vi "dfd_2-band Filter Bank Param Validation.vi"(4 "fs in [Hz]":dbl=800.0, 6 "weight":dbl=0.5, 7 "phase option":u16(ring) items=["Min-Max Phase", "Linear Phase"], 8 "error in (no error)":errorcluster, 9 "stopband attenuation [dB]":dbl=60.0, 10 "roll off":dbl=0.2, 11 "order":i32=38) -> (0 "error out":errorcluster, 1 "dup stopband attenuation [dB]":dbl=60.0, 2 "dup roll off":dbl, 3 "dup order":i32)   [LabVIEW 2017, in "NI_DigFilter_FilterBank.lvlib"]
doc: "Validates the parameters for the prototype filter design. If any parameter is not in their range, this VI will give an error report. If the order is not an integer of 2kM this VI will give a warning report, where k is any positive integer, and M is specified by <B>number of bands</B>."
uses:
  <vilib>/addons/Digital Filter Design/NI_DigFilter_FilterBank.lvlib
  <vilib>/addons/Digital Filter Design/_Misc.llb/dfd_Error Handlers (Multiple).vi
  <vilib>/addons/Digital Filter Design/NI_DigFilterLicensed.lvlib
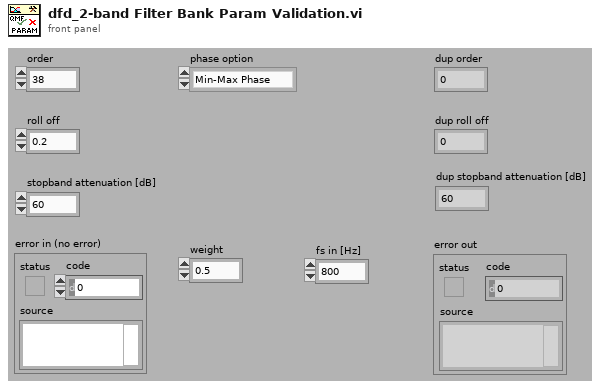
[diagram p1: front panel]
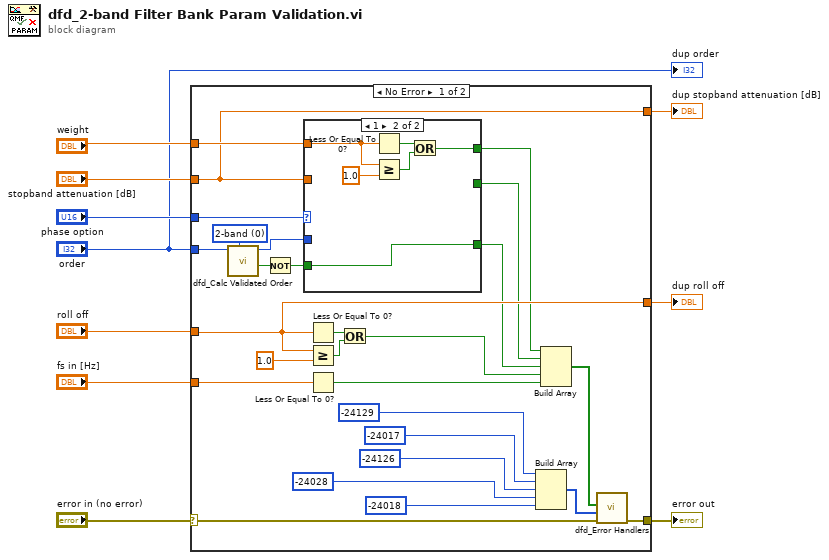
[diagram p0: block diagram]
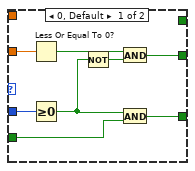
[diagram p2: hidden frame]
diagram:
  n1 = case shown="No Error" "error in (no error)" {
    selector: "error in (no error)" -> [w30 w52]
    tunnel: "order" -> [w15 _]
    tunnel: "roll off" -> [w33 _]
    tunnel: "weight" -> [w27 _]
    tunnel: [w35 w52] -> w8
    tunnel: [w33 _] -> w6
    tunnel: "phase option" -> [w28 _]
    tunnel: "stopband attenuation [dB]" -> [w25 _]
    tunnel: [w25 _] -> w3
    tunnel: "fs in [Hz]" -> [w18 _]
    frame No Error {
      w14 = u16 0 items=["2-band", "M-band Cosine-modulated PR"] ("bank type")
      n2 = call <vilib>:"dfd_Calc Validated Order.vi"("bank type"=w14, "order"=w15) -> ("valid?"=w12:bool, "dup order"=w13:i32)  [unwired: 7 in, 1 out]
      n3 = Not(x=w12) -> (.not. x?=w11:bool)
      n4 = case shown="1" w28 {
        tunnel: w13 -> [w39 _]
        tunnel: w25 -> [w45 _]
        tunnel: w27 -> [_ w48]
        tunnel: [_ w47] -> w26
        tunnel: [w42 _] -> w19
        tunnel: [w41 w46] -> w23
        tunnel: w11 -> [w38 w46]
        frame 0, Default {
          n5 = Less Or Equal To 0?(x=w45) -> (x <= 0?=w43:bool)
          n6 = Greater Or Equal To 0?(x=w39) -> (x >= 0?=w40:bool)
          n7 = Not(x=w40) -> (.not. x?=w44:bool)
          n8 = And(x=w43, y=w44) -> (x .and. y?=w42:bool)
          n9 = And(x=w40, y=w38) -> (x .and. y?=w41:bool)
        }
        frame 1 {
          n10 = Less Or Equal To 0?(x=w48) -> (x <= 0?=w50:bool)
          n11 = Greater Or Equal?(x=w48, y=1.0) -> (x >= y?=w51:bool)
          n12 = Or(x=w50, y=w51) -> (x .or. y?=w47:bool)
        }
      }
      n13 = Less Or Equal To 0?(x=w33) -> (x <= 0?=w34:bool)
      n14 = Greater Or Equal?(x=w33, y=1.0) -> (x >= y?=w32:bool)
      n15 = Less Or Equal To 0?(x=w18) -> (x <= 0?=w17:bool)
      n16 = Or(x=w34, y=w32) -> (x .or. y?=w21:bool)
      n17 = Build Array(-24129 ("ERR_INVALID_WEIGHT"), -24017 ("ERR_dB_LE_ZERO"), -24126 ("ERR_ORDER_EVEN"), -24028 ("ERR_ROLLOFF_RANGE_WRONG"), -24018 ("ERR_FS_LE_ZERO")) -> (w36:i32[])
      n18 = Build Array(w26, w19, w23, w21, w17) -> (w37:bool[])
      n19 = call-poly <vilib>:"dfd_Error Handlers.vi"("error in (no error)"=w30, "error sources"=w36, "condition failed?"=w37) -> ("error out"=w35:errorcluster)  [unwired: 8 in]
    }
    frame Error {
    }
  }
  "error out" <- w8
  "dup roll off" <- w6
  "dup stopband attenuation [dB]" <- w3
  "dup order" <- "order"
